vi "Get Invalid Chars.vi"() -> (2 "invalid chars":string[](array[string]))   [LabVIEW 2013, in "JUnit XML Tests.lvlib"]
doc: "Returns a list of characters that are invalid according to the XML specification."
uses:
  JUnit XML Tests.lvlib
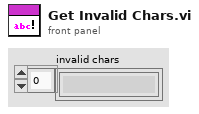
[diagram p1: front panel]
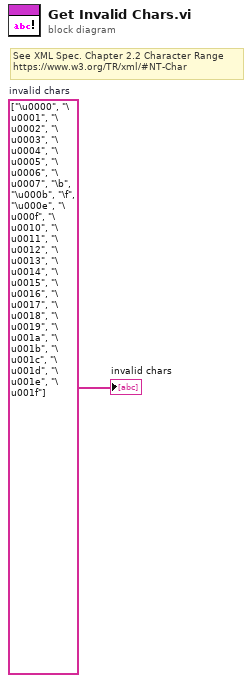
[diagram p0: block diagram]
diagram:
  w1 = string[] ["\u0000", "\u0001", "\u0002", "\u0003", "\u0004", "\u0005", "\u0006", "\u0007", "\b", "\u000b", "\f", "\u000e", "\u000f", "\u0010", "\u0011", "\u0012", "\u0013", "\u0014", "\u0015", "\u0016", "\u0017", "\u0018", "\u0019", "\u001a", "\u001b", "\u001c", "\u001d", "\u001e", "\u001f"]  # invalid chars
  # "See XML Spec. Chapter 2.2 Character Range\nhttps://www.w3.org/TR/xml/#NT-Char"
  "invalid chars" <- w1
